vi "Enter.vi"   [LabVIEW 2017]
uses:
  widgets/EnumStateMachine.llb/Main_Enum.ctl
  widgets/SP_tools.llb/Func_UIchange.ctl
  Controls/FV_Daqmx config.ctl
  widgets/EnumStateMachine.llb/Main_InsertQueue.vi
  widgets/EnumStateMachine.llb/Main_RemoveQueue.vi
  <vilib>/ErrorRing/Error Ring.xnode
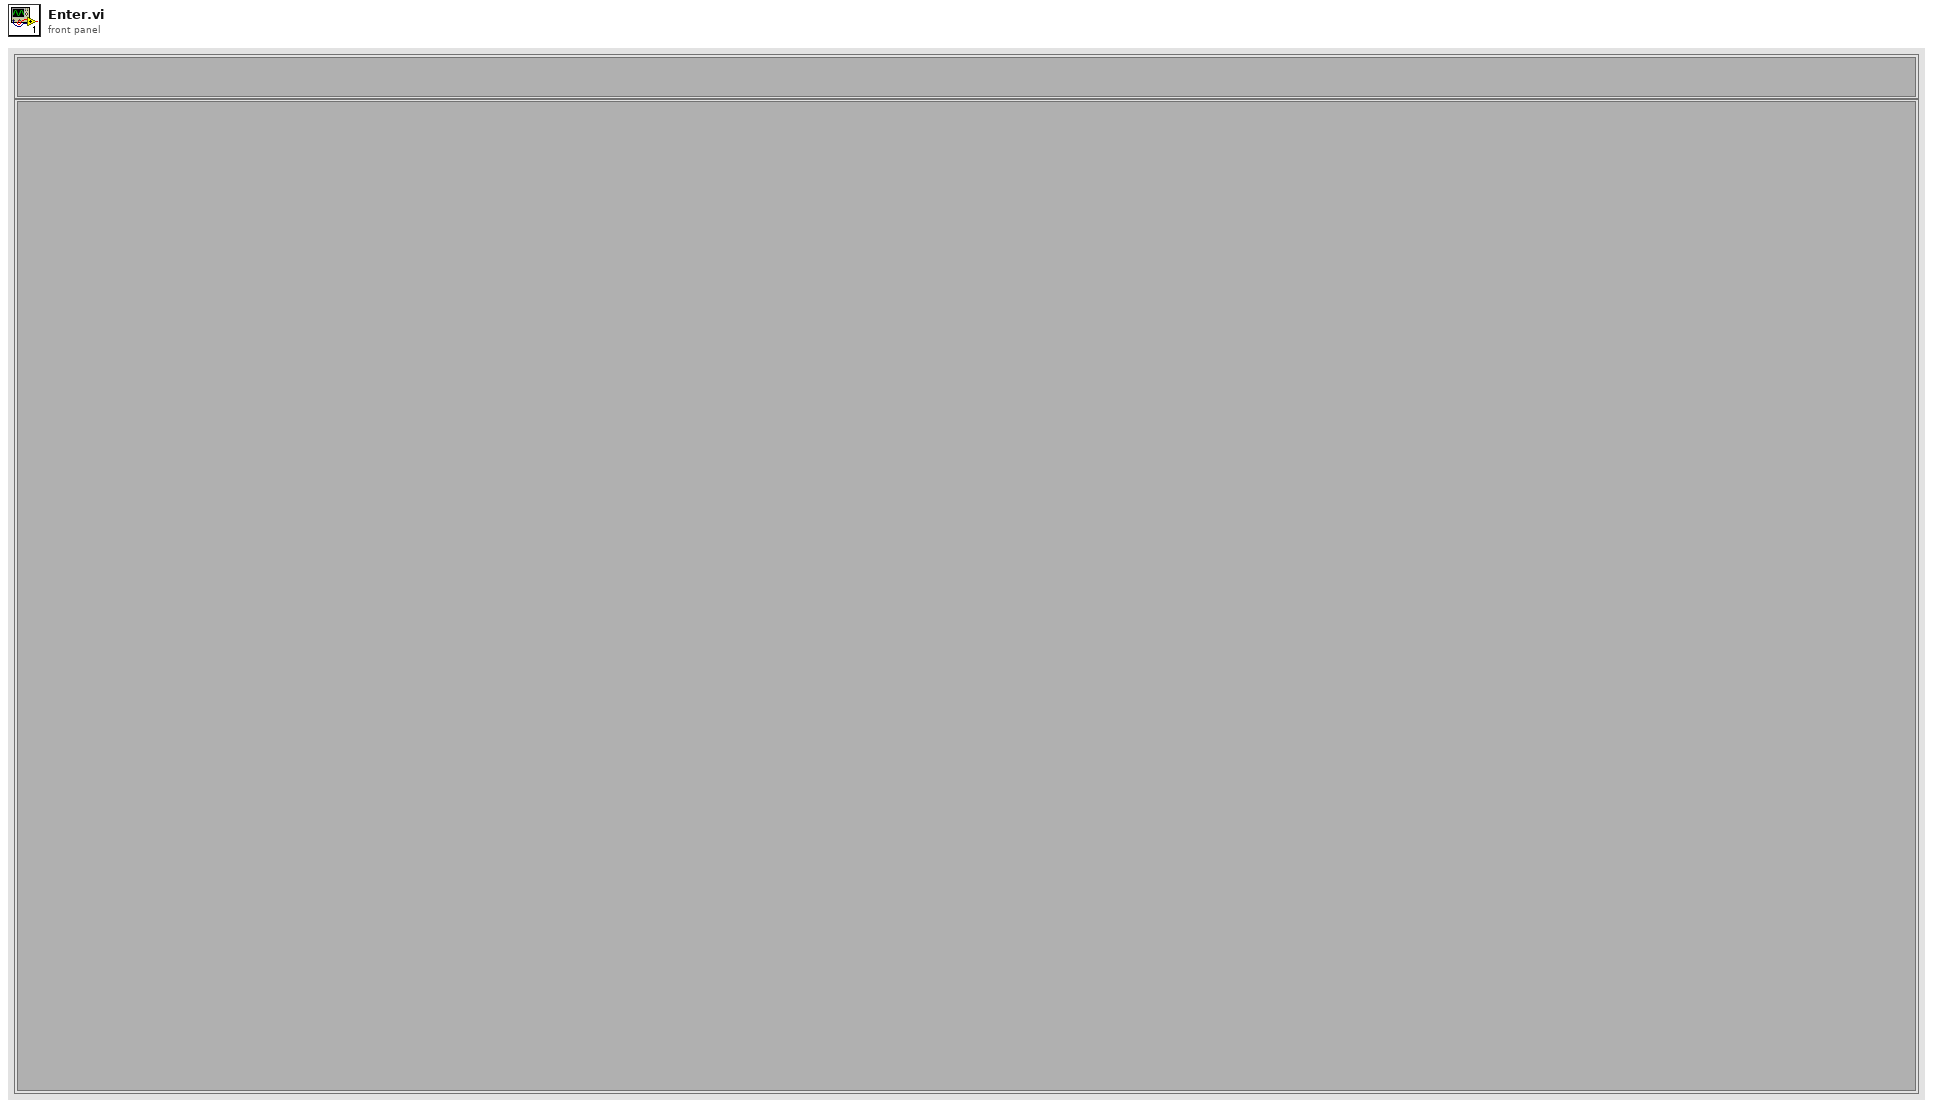
[diagram p1: front panel]
types:
  T1 = typedef "Main_Enum.ctl" = enum16{"Initialize", "SubPannel: Initialize", "Idel", "Show_Task infor", "Show_Daq config", "Run_Task", "Stop_Task", "Show_Alarm", "Show_Right", "Set_Save data", "Error handle", "Exit"}
  T2 = typedef "Queue RefNum" = refnum<k1>
  T3 = typedef "FV_Daqmx config.ctl" = enum16{"Initialize", "SetDefault", "UI_input", "GetAI", "GetCO", "GetCI"}
  T4 = typedef "Func_UIchange.ctl" = enum16{"Initialize", "Load Modules", "SP_Default", "SP_Replace", "Unload Modules"}
  T5 = cluster{"Image":path, "Modules":path, "System.ini":path}
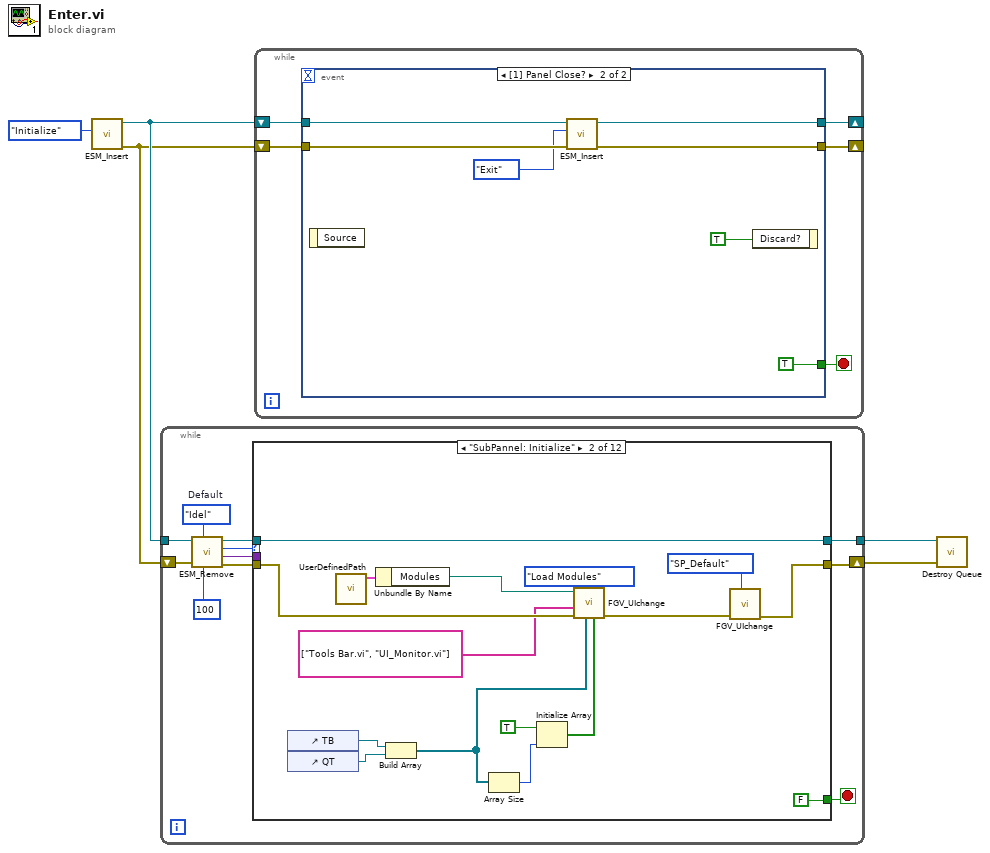
[diagram p0: block diagram]
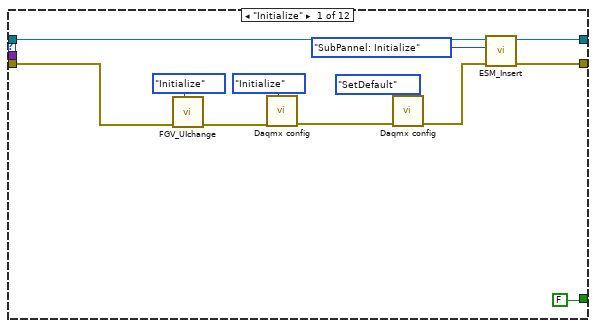
[diagram p2: hidden frame]
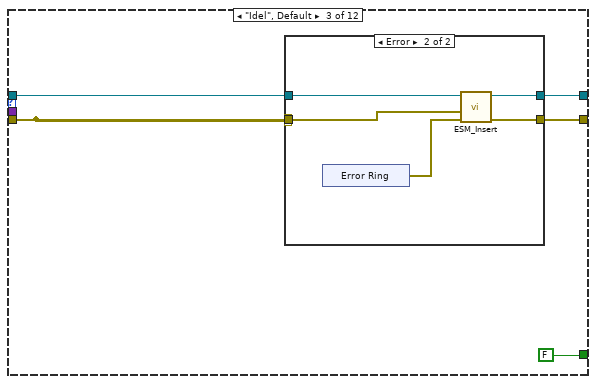
[diagram p3: hidden frame]
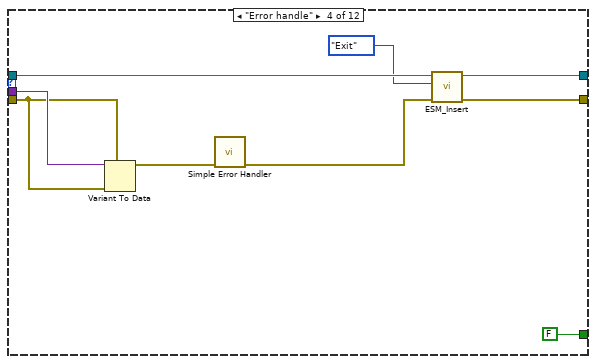
[diagram p5: hidden frame]
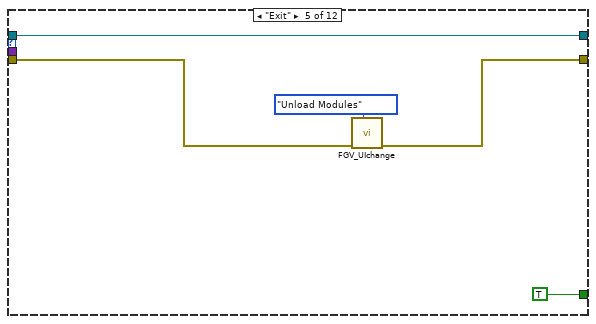
[diagram p6: hidden frame]
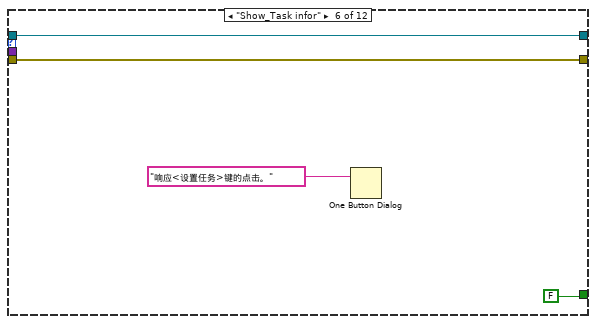
[diagram p7: hidden frame]
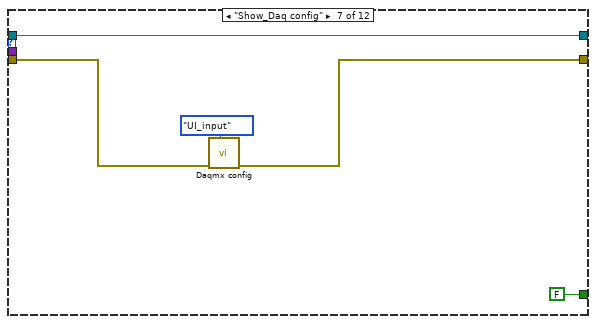
[diagram p8: hidden frame]
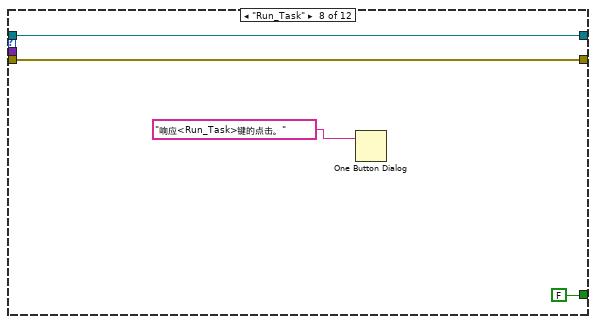
[diagram p9: hidden frame]
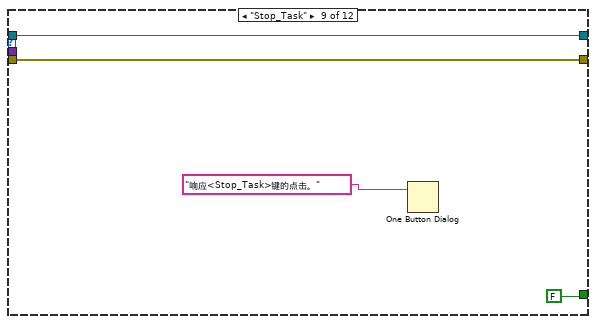
[diagram p10: hidden frame]
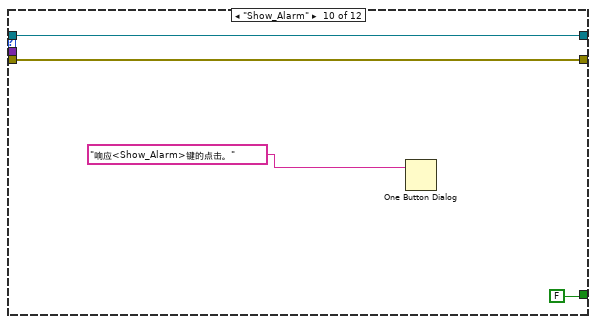
[diagram p11: hidden frame]
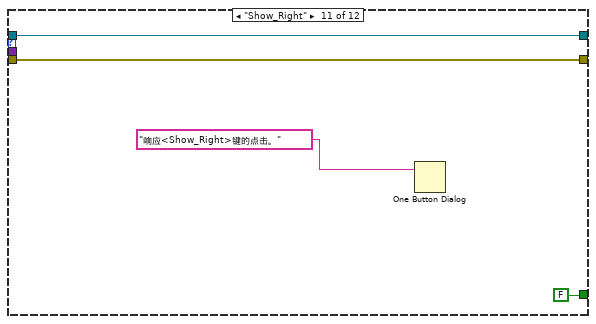
[diagram p12: hidden frame]
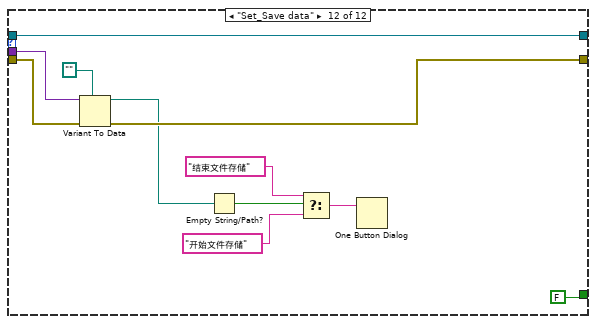
[diagram p13: hidden frame]
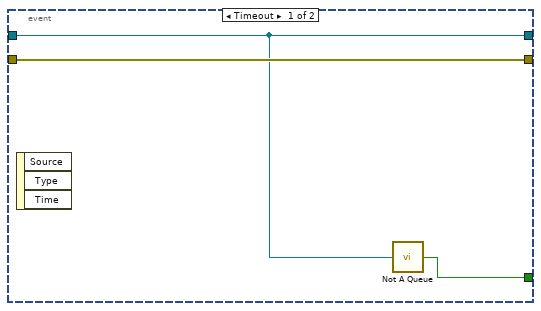
[diagram p14: hidden frame]
diagram:
  n1 = call-poly "ESM_Insert.vi"("Main"=Main_Enum."Initialize") -> ("error out"=w3:errorcluster, "queue out"=w4:T2)  [unwired: 9 in]
  n2 = while {
    tunnel: w4 -> [w16]
    shift-right: [w11] -> w1
    shift-left: w3 -> [w15]
    tunnel: [w7] -> w2
    stop <- w10 stop-if-true
    w6 = Main_Enum."Idel"  # Default
    n3 = call-poly "ESM_Remove.vi"("ms timeout (-1)"=100, "Default"=w6, "error in (no error)"=w15, "queue"=w16) -> ("错误输出"=w13:errorcluster, "data"=w9:variant, "Main"=w14:T1, "queue out"=w12:T2)  [unwired: 4 in]
    n4 = case shown="\"SubPannel: Initialize\"" w14 {
      tunnel: w13 -> [w23 w44 w45 w64 w71 w74 w77 w83 w87 w91 w95 w106]
      tunnel: w12 -> [w28 w41 w49 w62 w69 w75 w79 w84 w88 w92 w96 w107]
      tunnel: [w26 w43 w48 w59 w68 w74 w76 w83 w87 w91 w95 w103] -> w11
      tunnel: [FALSE FALSE FALSE FALSE TRUE FALSE FALSE FALSE FALSE FALSE FALSE FALSE] -> w10
      tunnel: w9 -> [_ _ _ w65 _ _ _ _ _ _ _ w105]
      tunnel: [w24 w41 w46 w61 w69 w75 w79 w84 w88 w92 w96 w107] -> w7
      frame "Initialize" {
        n5 = call "FGV_UIchange.vi"("FV_UIchange"=Func_UIchange."Initialize", "error in (no error)"=w23) -> ("error out"=w20:errorcluster)  [unwired: 8 in, 1 out]
        n6 = call "Daqmx config.vi"("FV"=FV_Daqmx_config."Initialize", "error in (no error)"=w20) -> ("error out"=w19:errorcluster)  [unwired: 6 in, 3 out]
        n7 = call "Daqmx config.vi"("FV"=FV_Daqmx_config."SetDefault", "error in (no error)"=w19) -> ("error out"=w17:errorcluster)  [unwired: 6 in, 3 out]
        n8 = call-poly "ESM_Insert.vi"("error in (no error)"=w17, "Main"=Main_Enum."SubPannel: Initialize", "queue"=w28) -> ("error out"=w26:errorcluster, "queue out"=w24:T2)  [unwired: 7 in]
      }
      frame "SubPannel: Initialize" {
        n9 = control-ref of="TB"() -> (w31:refnum<vi>)
        n10 = control-ref of="QT"() -> (w32:refnum<vi>)
        n11 = call "UserDefinedPath.vi"() -> ("ProDefPath"=w39:T5)  [unwired: 11 in]
        n12 = Unbundle By Name(w39) -> ("Modules"=w38:path)
        n13 = Build Array(w31, w32) -> (w30:refnum<vi>[])
        n14 = Array Size(array=w30) -> (size(s)=w29:i32)
        n15 = Initialize Array(TRUE, w29) -> (w33:bool[])
        n16 = call "FGV_UIchange.vi"("Running"=w33, "SP_refre"=w30, "FV_UIchange"=Func_UIchange."Load Modules", "error in (no error)"=w44, "Modules"=string[] ["Tools Bar.vi", "UI_Monitor.vi"], "ModulesPath"=w38) -> ("error out"=w36:errorcluster)  [unwired: 4 in, 1 out]
        n17 = call "FGV_UIchange.vi"("FV_UIchange"=Func_UIchange."SP_Default", "error in (no error)"=w36) -> ("error out"=w43:errorcluster)  [unwired: 8 in, 1 out]
      }
      frame "Idel", Default {
        n18 = case shown="Error" w45 {
          tunnel: w49 -> [w51 w56]
          tunnel: [w50 w54] -> w48
          tunnel: w45 -> [w50 w53]
          tunnel: [w51 w52] -> w46
          frame No Error {
          }
          frame Error {
            n19 = xnode "Error Ring"() -> ("error out"=w55:errorcluster)
            n20 = call-poly "ESM_Insert.vi"("error in (no error)"=w55, "data"=w53, "queue"=w56) -> ("error out"=w54:errorcluster, "queue out"=w52:T2)  [unwired: 7 in]
          }
        }
      }
      frame "Error handle" {
        n21 = Variant To Data(error in=w64, type=w64, Variant=w65) -> (data=w63:errorcluster)  [unwired: 1 out]
        n22 = call <vilib>:"Simple Error Handler.vi"("error in (no error)"=w63) -> ("error out"=w60:errorcluster)  [unwired: 4 in, 4 out]
        n23 = call-poly "ESM_Insert.vi"("error in (no error)"=w60, "Main"=Main_Enum."Exit", "queue"=w62) -> ("error out"=w59:errorcluster, "queue out"=w61:T2)  [unwired: 7 in]
      }
      frame "Exit" {
        n24 = call "FGV_UIchange.vi"("FV_UIchange"=Func_UIchange."Unload Modules", "error in (no error)"=w71) -> ("error out"=w68:errorcluster)  [unwired: 8 in, 1 out]
      }
      frame "Show_Task infor" {
        n25 = One Button Dialog(message="响应<设置任务>键的点击。") -> ()  [unwired: 1 in, 1 out]
      }
      frame "Show_Daq config" {
        n26 = call "Daqmx config.vi"("FV"=FV_Daqmx_config."UI_input", "error in (no error)"=w77) -> ("error out"=w76:errorcluster)  [unwired: 6 in, 3 out]
      }
      frame "Run_Task" {
        n27 = One Button Dialog(message="响应<Run_Task>键的点击。") -> ()  [unwired: 1 in, 1 out]
      }
      frame "Stop_Task" {
        n28 = One Button Dialog(message="响应<Stop_Task>键的点击。") -> ()  [unwired: 1 in, 1 out]
      }
      frame "Show_Alarm" {
        n29 = One Button Dialog(message="响应<Show_Alarm>键的点击。") -> ()  [unwired: 1 in, 1 out]
      }
      frame "Show_Right" {
        n30 = One Button Dialog(message="响应<Show_Right>键的点击。") -> ()  [unwired: 1 in, 1 out]
      }
      frame "Set_Save data" {
        n31 = Variant To Data(error in=w106, type=path "", Variant=w105) -> (data=w101:path, error out=w103:errorcluster)
        n32 = Empty String/Path?(string/path=w101) -> (empty?=w100:bool)
        n33 = Select(t="结束文件存储", s=w100, f="开始文件存储") -> (s? t:f=w98:string)
        n34 = One Button Dialog(message=w98) -> ()  [unwired: 1 in, 1 out]
      }
    }
  }
  n35 = while {
    shift-right: [w109] -> _
    shift-left: w4 -> [w111]
    shift-right: [w108] -> _
    shift-left: w3 -> [w110]
    stop <- w112 stop-if-true
    n36 = event shown="[1] Panel Close?" {
      selector: _ -> [_ _]
      dyn-events: _ -> [_ _]
      timeout: _ -> [_ _]
      tunnel: [w113 TRUE] -> w112
      tunnel: [w114 w119] -> w109
      tunnel: w111 -> [w114 w121]
      tunnel: [w115 w117] -> w108
      tunnel: w110 -> [w115 w118]
      event Timeout {
        n37 = event-data() -> ()  [unwired: 1 in, 3 out]
        n38 = call <vilib>:"Not A Queue.vi"("queue"=w114) -> ("is a queue?"=w113:bool)
      }
      event Panel Close? {
        n39 = event-data() -> ()  [unwired: 1 in, 1 out]
        n40 = call-poly "ESM_Insert.vi"("error in (no error)"=w118, "Main"=Main_Enum."Exit", "queue"=w121) -> ("error out"=w117:errorcluster, "queue out"=w119:T2)  [unwired: 7 in]
        n41 = event-data("Discard?"=TRUE) -> ()  [unwired: 1 in, 1 out]
      }
    }
  }
  n42 = call <vilib>:"Destroy Queue.vi"("error in (no error)"=w1, "queue"=w2) -> ()  [unwired: 3 in, 3 out]
